vi "Search_and_match2.vi"(0 "Learn Mode":u32(ring)=1 items=["All", "Shift Information", "Rotation Information"], 1 "Feature Mode":u32(ring) items=["Color and Shape", "Color", "Shape "], 2 "Minimum Match Score":sgl=800.0 min=0 max=1000 format="%.2f", 3 "Number of Matches Requested":i32=1 min=1, 4 "Match Mode":u32(ring) items=["Shift Invariant", "Rotation Invariant"], 6 "Ref path":path, 7 "Match Feature Mode":u32(ring)=2 items=["Color and Shape", "Color", "Shape"], 8 "Main Path":path) -> (12 "Match values":T4, 14 "Number of Matches":i32, 15 "Total Score":sgl, 16 "Shape Score":sgl, 17 "Main Image":T2(plugin-control))   [LabVIEW 2025]
uses:
  <vilib>/vision/NI_Vision_Development_Module.lvlib
panel:
  in  "White with color":bool
  out "Fail 2?":bool
  out "Particle Reports (Pixels) 2":T1(array[cluster]) {"Orientation" format="%.2f"; "Dimensions"."Height" format="%.2f"; "Dimensions"."Width" format="%.2f"; "Center of Mass"."Y" format="%.2f"; "Center of Mass"."X" format="%.2f"; "Bounding Rect"."Bottom" format="%.2f"; "Bounding Rect"."Right" format="%.2f"; "Bounding Rect"."Top" format="%.2f"; "Bounding Rect"."Left" format="%.2f"; "Number of Holes" format="%.2f"; "Area" format="%.2f"}
  out "Image 3":T2(plugin-control)
  out "Number of Particles 2":i32
  out "Histogram Report 2":T3 {"Standard  Variation" format="%.2f"; "Mean Value" format="%.2f"; "Interval Width" format="%.2f"; "Starting Value" format="%.2f"; "Maximal Value" format="%.2f"; "Minimal Value" format="%.2f"}
  out "Image":T2(plugin-control)
  in  "Match Mode 2":u32(ring) items=["Shift Invariant", "Rotation Invariant"]
  in  "Match Feature Mode 2":u32(ring)=1 items=["Color and Shape", "Color", "Shape"]
  in  "Rotation Angle Ranges (degrees) 2":cluster{sgl, sgl}[](array[cluster]) {"?" format="%.2f"; "?" format="%.2f"}
  out "Match values 2":T4
  out "Matches 2":T5(array[cluster]) {"Bounding Box"."y" format="%.2f"; "Bounding Box"."x" format="%.2f"; "Position"."y" format="%.2f"; "Position"."x" format="%.2f"; "Score" format="%.2f"; "Scale" format="%.2f"; "Angle" format="%.2f"}
  out "error out":errorcluster
  out "Extraced_Image":T2(plugin-control)
  in  "Rotation Angle Ranges (degrees)":cluster{sgl, sgl}[](array[cluster]) {"?" format="%.2f"; "?" format="%.2f"}
  out "Ref image":T2(plugin-control)
  out "Matches":T5(array[cluster]) {"Bounding Box"."y" format="%.2f"; "Bounding Box"."x" format="%.2f"; "Position"."y" format="%.2f"; "Position"."x" format="%.2f"; "Score" format="%.2f"; "Scale" format="%.2f"; "Angle" format="%.2f"}
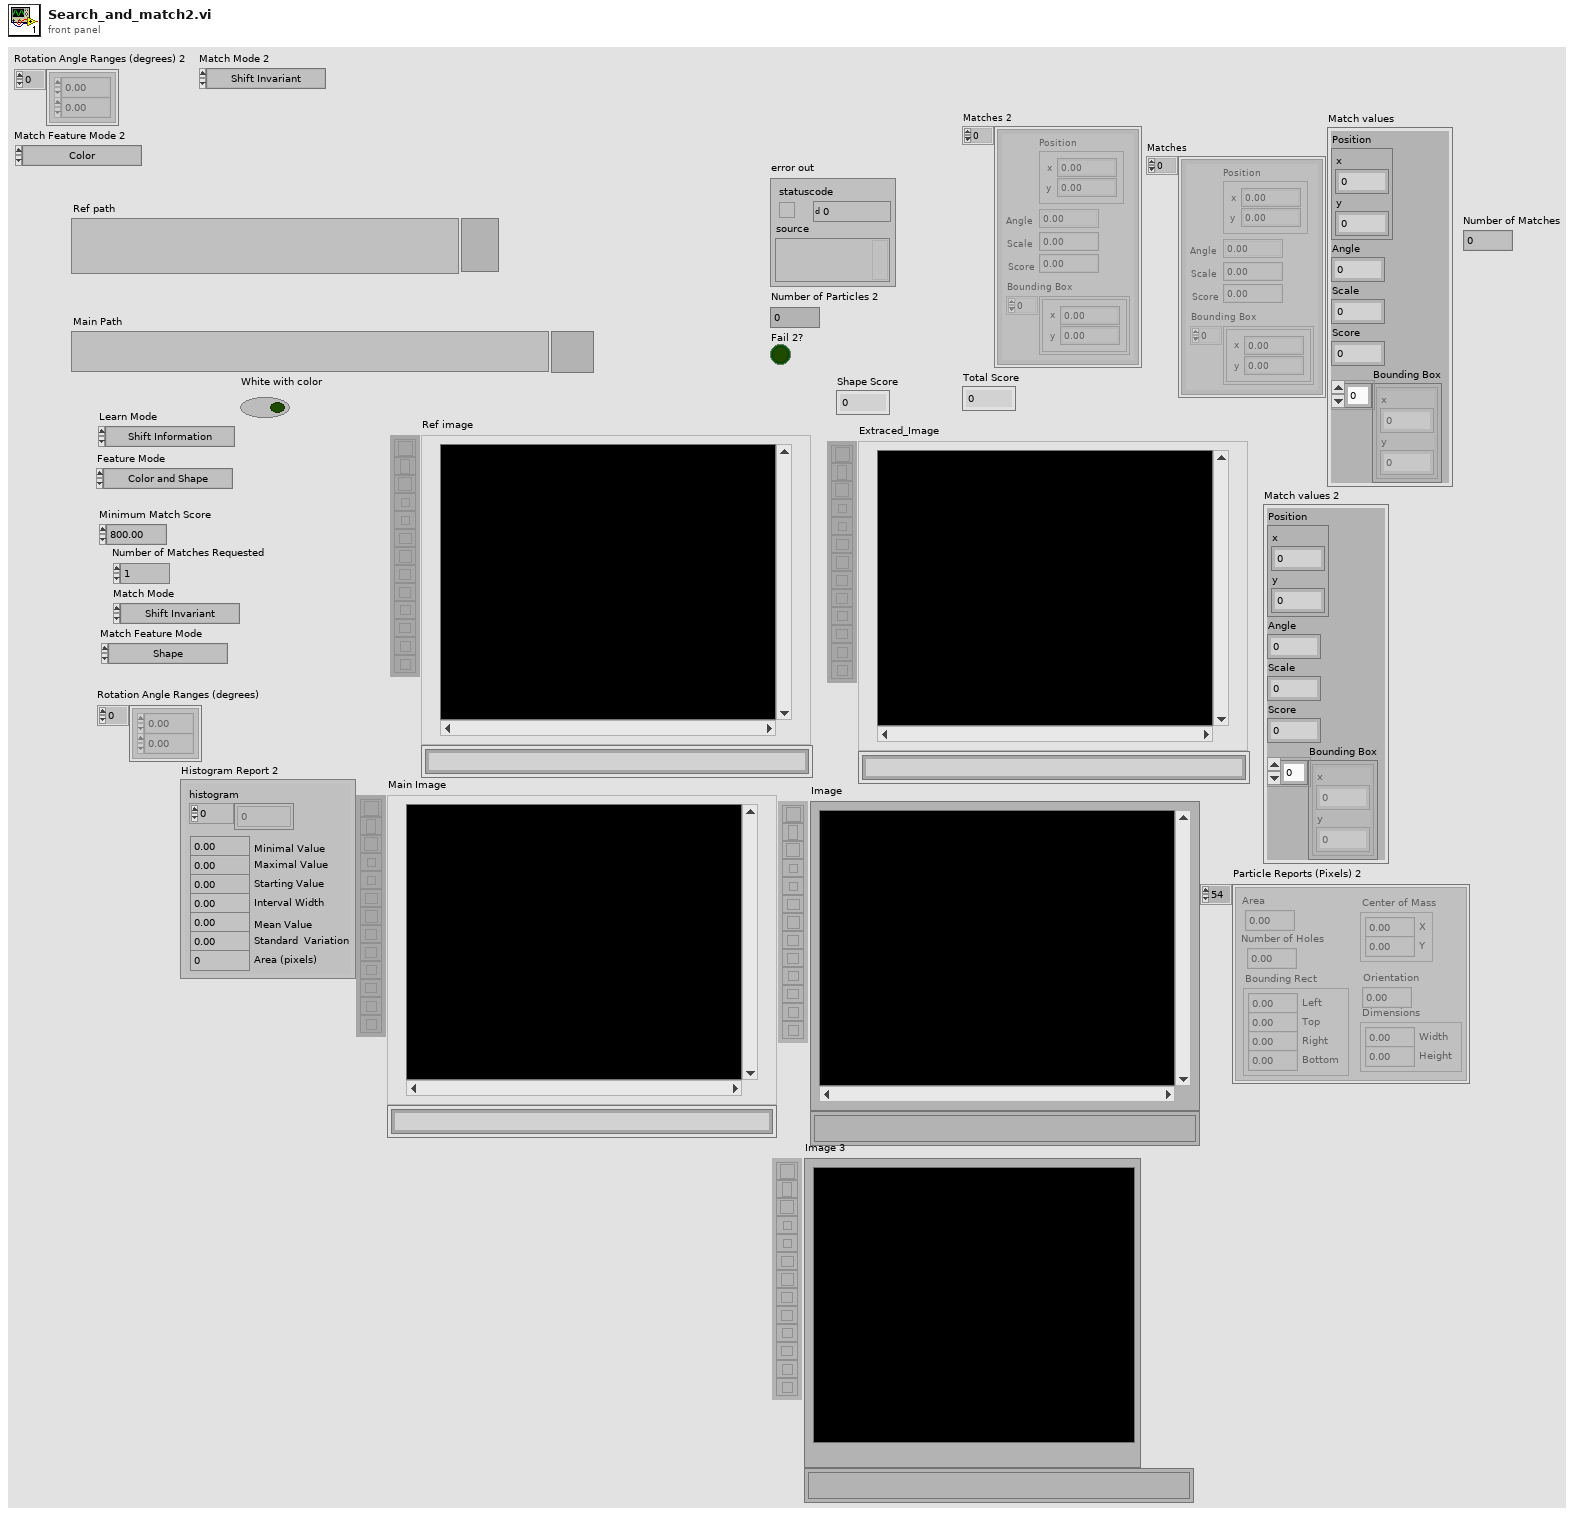
[diagram p1: front panel]
types:
  T1 = cluster{"Area":dbl, "Number of Holes":dbl, "Bounding Rect":cluster{"Left":dbl, "Top":dbl, "Right":dbl, "Bottom":dbl}, "Center of Mass":cluster{"X":dbl, "Y":dbl}, "Orientation":dbl, "Dimensions":cluster{"Width":dbl, "Height":dbl}}[]
  T2 = typedef "IMAQ Image.ctl" = refnum<image>
  T3 = cluster{"histogram":u32[], "Minimal Value":sgl, "Maximal Value":sgl, "Starting Value":sgl, "Interval Width":sgl, "Mean Value":sgl, "Standard  Variation":sgl, "Area (pixels)":i32}
  T4 = cluster{"Position":cluster{"x":sgl, "y":sgl}, "Angle":sgl, "Scale":sgl, "Score":sgl, "Bounding Box":cluster{"x":sgl, "y":sgl}[]}
  T5 = cluster{"Position":cluster{"x":sgl, "y":sgl}, "Angle":sgl, "Scale":sgl, "Score":sgl, "Bounding Box":cluster{"x":sgl, "y":sgl}[]}[]
  T6 = typedef "Image Type" = u32
  T7 = typedef "IMAQ Rectangle" = cluster{"Left":i32, "Top":i32, "Right":i32, "Bottom":i32, "Rotation":dbl}
  T8 = typedef "ROI Descriptor" = cluster{"Global Rectangle":i32[], "Contours":cluster{"ID":enum32{"External", "Internal"}, "Type":u32, "Coordinates":i32[]}[]}
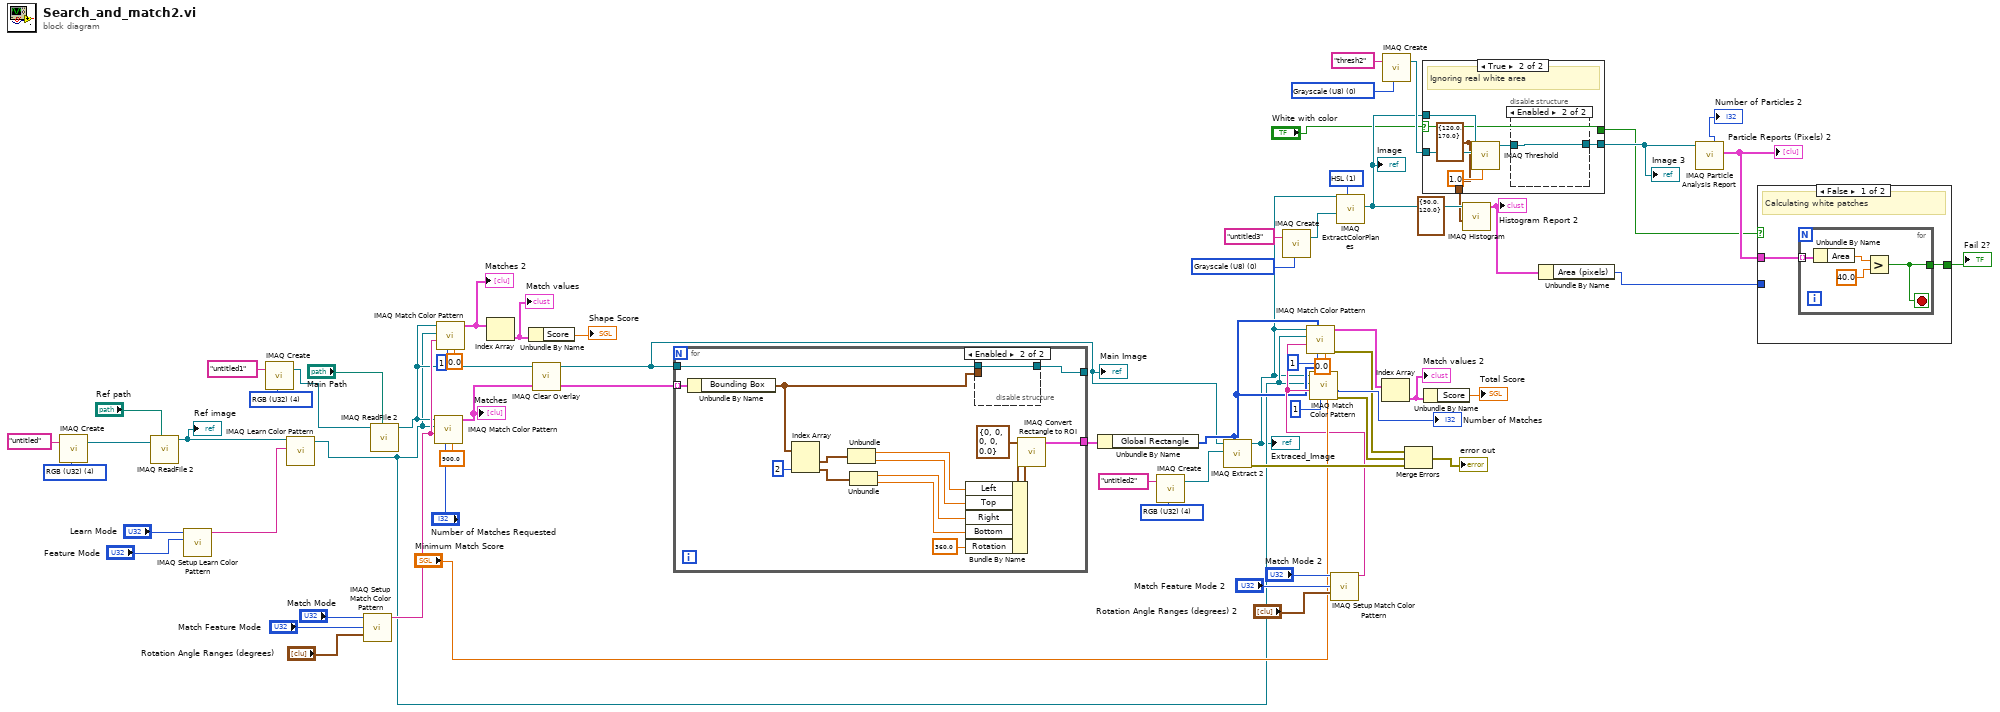
[diagram p0: block diagram]
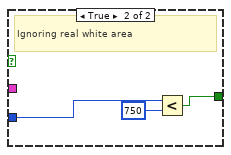
[diagram p2: hidden frame]
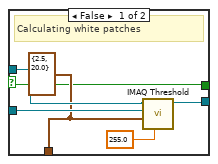
[diagram p3: hidden frame]
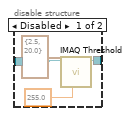
[diagram p4: hidden frame]
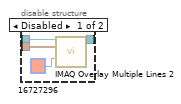
[diagram p5: hidden frame]
diagram:
  w14 = T6 0 items=["Grayscale (U8)", "Grayscale (I16)", "Grayscale (SGL)", "Complex (CSG)", "RGB (U32)", "HSL (U32)", "RGB (U64)", "Grayscale (U16)"] ("Image Type")
  (unwired) cluster{"Minimum":sgl, "Maximum":sgl} {"Minimum"=90.0, "Maximum"=120.0} ("Interval Range")
  w18 = u16 1 items=["RGB", "HSL", "HSV", "HSI"] ("Color Mode")
  w16 = T6 0 items=["Grayscale (U8)", "Grayscale (I16)", "Grayscale (SGL)", "Complex (CSG)", "RGB (U32)", "HSL (U32)", "RGB (U64)", "Grayscale (U16)"] ("Image Type")
  w51 = T6 4 items=["Grayscale (U8)", "Grayscale (I16)", "Grayscale (SGL)", "Complex (CSG)", "RGB (U32)", "HSL (U32)", "RGB (U64)", "Grayscale (U16)"] ("Image Type")
  w62 = T6 4 items=["Grayscale (U8)", "Grayscale (I16)", "Grayscale (SGL)", "Complex (CSG)", "RGB (U32)", "HSL (U32)", "RGB (U64)", "Grayscale (U16)"] ("Image Type")
  w65 = T6 4 items=["Grayscale (U8)", "Grayscale (I16)", "Grayscale (SGL)", "Complex (CSG)", "RGB (U32)", "HSL (U32)", "RGB (U64)", "Grayscale (U16)"] ("Image Type")
  n1 = call "IMAQ Create"("Image Name"="untitled", "Image Type"=w65) -> ("New Image"=w64:T2)  [unwired: 3 in, 1 out]
  n2 = call "IMAQ ReadFile 2"("File Path"="Ref path", "Image"=w64) -> ("Image Out"=w53:T2)  [unwired: 5 in, 4 out]
  "Ref image" <- w53
  n3 = call "IMAQ Setup Learn Color Pattern"("Feature Mode"="Feature Mode", "Learn Mode"="Learn Mode") -> ("Learn Color Pattern Setup Data"=w58:string)  [unwired: 8 in, 1 out]
  n4 = call "IMAQ Create"("Image Name"="untitled1", "Image Type"=w62) -> ("New Image"=w57:T2)  [unwired: 3 in, 1 out]
  n5 = call "IMAQ Learn Color Pattern"("Learn Color Pattern Setup Data"=w58, "Image"=w53) -> ("Template Image Out"=w19:T2)  [unwired: 8 in, 1 out]
  n6 = call "IMAQ Setup Match Color Pattern"("Match Mode"="Match Mode", "Match Feature Mode"="Match Feature Mode", "Rotation Angle Ranges (degrees)"="Rotation Angle Ranges (degrees)") -> ("Match Color Pattern Setup Data"=w47:string)  [unwired: 11 in, 1 out]
  n7 = call "IMAQ ReadFile 2"("File Path"="Main Path", "Image"=w57) -> ("Image Out"=w25:T2)  [unwired: 5 in, 4 out]
  n8 = call "IMAQ Match Color Pattern"("Minimum Match Score"=sgl 900.0, "Number of Matches Requested"="Number of Matches Requested", "Match Color Pattern Setup Data"=w47, "Template Image"=w19, "Image"=w25) -> ("Matches"=w37:T5)  [unwired: 4 in, 2 out]
  "Matches" <- w37
  n9 = call "IMAQ Match Color Pattern"("Minimum Match Score"=sgl 0.0, "Number of Matches Requested"=1, "Match Color Pattern Setup Data"=w47, "Template Image"=w19, "Image"=w25) -> ("Matches"=w44:T5)  [unwired: 4 in, 2 out]
  "Matches 2" <- w44
  n10 = Index Array(array=w44) -> (element=w43:T4)  [unwired: 1 in]
  "Match values" <- w43
  n11 = Unbundle By Name(w43) -> ("Score"=→"Shape Score":sgl)
  n12 = call "IMAQ Clear Overlay"("Image"=w25) -> ("Image Out"=w21:T2)  [unwired: 9 in, 1 out]
  "Main Image" <- w21
  n13 = for {
    tunnel: w21 -> [w81]
    tunnel: w37 -> [w80] mode=indexing
    tunnel: [w79] -> _
    tunnel: [w68] -> w20
    n14 = Unbundle By Name(w80) -> ("Bounding Box"=w75:cluster{"x":sgl, "y":sgl}[])
    n15 = Index Array(array=w75, index #2=2 ("index")) -> (element #1=w74:cluster{"x":sgl, "y":sgl}, element #2=w73:cluster{"x":sgl, "y":sgl})  [unwired: 1 in]
    n16 = Unbundle(w74) -> ("x"=w72:sgl, "y"=w71:sgl)
    n17 = Unbundle(w73) -> ("x"=w70:sgl, "y"=w69:sgl)
    n18 = Bundle By Name(cluster=T7 {"Left"=0, "Top"=0, "Right"=0, "Bottom"=0, "Rotation"=0.0} ("Rectangle"), "Left"=w72, "Top"=w71, "Right"=w70, "Bottom"=w69, "Rotation"=360.0) -> (w77:T7)
    n19 = disable-structure shown="Enabled" {
      disable-tunnel: w81 -> [w85 w86]
      disable-tunnel: [w83 w86] -> w79
      disable-tunnel: w75 -> [w82 _]
      frame Disabled {
        n20 = call "IMAQ Overlay Multiple Lines 2"("Image"=w85, "Line End Points"=w82, "Color"=u32 16727296) -> ("Image Out"=w83:T2)  [unwired: 11 in, 1 out]
      }
      frame Enabled {
      }
    }
    n21 = call "IMAQ Convert Rectangle to ROI"("Rectangle"=w77) -> ("ROI Descriptor"=w68:T8)  [unwired: 8 in, 1 out]
  }
  n22 = Unbundle By Name(w20) -> ("Global Rectangle"=w22:i32[])
  n23 = call "IMAQ Create"("Image Name"="untitled2", "Image Type"=w51) -> ("New Image"=w49:T2)  [unwired: 3 in, 1 out]
  n24 = call "IMAQ Extract 2"("Optional Rectangle"=w22, "Image Dst"=w49, "Image Src"=w21) -> ("error out"=w48:errorcluster, "Image Dst Out"=w1:T2)  [unwired: 7 in]
  "Extraced_Image" <- w1
  n25 = call "IMAQ Create"("Image Name"="untitled3", "Image Type"=w16) -> ("New Image"=w11:T2)  [unwired: 3 in, 1 out]
  n26 = call "IMAQ Setup Match Color Pattern"("Match Mode"="Match Mode 2", "Match Feature Mode"="Match Feature Mode 2", "Rotation Angle Ranges (degrees)"="Rotation Angle Ranges (degrees) 2") -> ("Match Color Pattern Setup Data"=w30:string)  [unwired: 11 in, 1 out]
  n27 = call "IMAQ Match Color Pattern"("Minimum Match Score"=sgl 0.0, "Number of Matches Requested"=1, "Optional Rectangle"=w22, "Match Color Pattern Setup Data"=w30, "Template Image"=w19, "Image"=w1) -> ("error out"=w26:errorcluster, "Matches"=w27:T5)  [unwired: 3 in, 1 out]
  n28 = call "IMAQ Match Color Pattern"("Minimum Match Score"="Minimum Match Score", "Number of Matches Requested"=1, "Optional Rectangle"=w22, "Match Color Pattern Setup Data"=w30, "Template Image"=w19, "Image"=w1) -> ("error out"=w35:errorcluster, "Number of Matches"=→"Number of Matches":i32)  [unwired: 3 in, 1 out]
  n29 = call "IMAQ ExtractColorPlanes"("Color Mode"=w18, "Green or Sat Plane"=w11, "Image Src"=w1) -> ("Green or Sat Plane out"=w10:T2)  [unwired: 5 in, 3 out]
  "Image" <- w10
  n30 = Index Array(array=w27) -> (element=w41:T4)  [unwired: 1 in]
  "Match values 2" <- w41
  n31 = call "IMAQ Create"("Image Name"="thresh2", "Image Type"=w14) -> ("New Image"=w12:T2)  [unwired: 3 in, 1 out]
  n32 = Merge Errors(w26, w35, w48) -> (→"error out":errorcluster)
  n33 = case shown="True" "White with color" {
    selector: "White with color" -> [w87 w93]
    tunnel: w12 -> [w90 w99]
    tunnel: w10 -> [w91 w98]
    tunnel: [w89 w96] -> w7
    tunnel: [w88 w94] -> w4
    tunnel: [w87 w93] -> w3
    frame False {
      w88 = cluster{"Lower value":sgl, "Upper value":sgl} {"Lower value"=2.5, "Upper value"=20.0} ("Range")
      # "Calculating white patches"
      n34 = call "IMAQ Threshold"("Replace Value"=sgl 255.0, "Range"=w88, "Image Dst"=w90, "Image Src"=w91) -> ("Image Dst Out"=w89:T2)  [unwired: 6 in, 1 out]
    }
    frame True {
      w94 = cluster{"Lower value":sgl, "Upper value":sgl} {"Lower value"=120.0, "Upper value"=170.0} ("Range")
      # "Ignoring real white area"
      n35 = call "IMAQ Threshold"("Replace Value"=sgl 1.0, "Range"=w94, "Image Dst"=w99, "Image Src"=w98) -> ("Image Dst Out"=w95:T2)  [unwired: 6 in, 1 out]
      n36 = disable-structure shown="Enabled" {
        disable-tunnel: [w101 w104] -> w96
        disable-tunnel: w95 -> [w100 w104]
        frame Disabled {
          n37 = call "IMAQ Threshold"("Replace Value"=sgl 255.0, "Range"=cluster{"Lower value":sgl, "Upper value":sgl} {"Lower value"=2.5, "Upper value"=20.0}, "Image Src"=w100) -> ("Image Dst Out"=w101:T2)  [unwired: 7 in, 1 out]
        }
        frame Enabled {
        }
      }
    }
  }
  "Image 3" <- w7
  n38 = Unbundle By Name(w41) -> ("Score"=→"Total Score":sgl)
  n39 = call "IMAQ Histogram"("Interval Range"=w4, "Image"=w10) -> ("Histogram Report"=w15:T3)  [unwired: 8 in, 1 out]
  "Histogram Report 2" <- w15
  n40 = Unbundle By Name(w15) -> ("Area (pixels)"=w2:i32)
  n41 = call "IMAQ Particle Analysis Report"("Image"=w7) -> ("Particle Reports (Pixels)"=w9:T1, "Number of Particles"=→"Number of Particles 2":i32)  [unwired: 5 in, 4 out]
  "Particle Reports (Pixels) 2" <- w9
  n42 = case shown="False" w3 {
    tunnel: w9 -> [w106 _]
    tunnel: [w105 w111] -> w8
    tunnel: w2 -> [_ w113]
    frame False {
      # "Calculating white patches"
      n43 = for {
        tunnel: w106 -> [w110] mode=indexing
        tunnel: [w107] -> w105
        stop <- w107 stop-if-true
        n44 = Unbundle By Name(w110) -> ("Area"=w108:dbl)
        n45 = Greater?(x=w108, y=40.0) -> (0:w107:bool)
      }
    }
    frame True {
      # "Ignoring real white area"
      n46 = Less?(x=w113, y=750) -> (x < y?=w111:bool)
    }
  }
  "Fail 2?" <- w8
